vi "Dashboard Main.vi"() -> ()   [LabVIEW 2015]
uses:
  vision/Camera Types.ctl
  <vilib>/Utility/miscctls.llb/LVRowAndColumnTypeDef.ctl
  <vilib>/event_ctls.llb/eventvkey.ctl
  <vilib>/Rock Robotics/WPI/Dashboard/WPI_DashboardLogging Global.vi
  <vilib>/Rock Robotics/Network Tables/NT Read Boolean.vi
  <vilib>/Utility/config.llb/Write Key (String).vi
  <vilib>/Utility/config.llb/Write Key (I32).vi
  <vilib>/Utility/config.llb/NI_LVConfig.lvlib
  Custom/BB_AutonomousSelector.lvlib
  <vilib>/vision/NI_Vision_Development_Module.lvlib
panel:
  in  "Camera Settings":T1={"Frame Rate"=30, "Compression"=30, "Size"=1} {"Frame Rate" scale=1.0..30.0; "Size" items=["640x480", "320x240", "160x120"]}
  in  "DB Camera Config":bool
  out "fps":dbl format="%#.1g"
  out "Mbps":dbl format="%#.1g"
  out "Mbps LED":bool
  out "fps":dbl format="%#.1g"
  out "Mbps 2":dbl format="%#.1g"
  out "Mbps LED 2":bool
  out "Camera Image 2":T2(plugin-control)
  out "Camera Image":T2(plugin-control)
  out "Camera IP 2":string
  in  "TCP":refnum<k5>
  in  "Rec Mode":enum32{"Stop", "Record", "Playback"}(radio)
  in  "Vision":u16(ring) items=["Camera Off", "USB Camera SW", "USB Camera HW", "IP Camera"]
  out "USB Camera IP":string
  out "Image Message":string="Timeout in Camera Communications"
  in  "Dashboard Tab":T3(tab)
  in  "Obstacle":u16(ring) items=["Mars Rock", "BETA_1BALL_STRAIGHT", "BETA_1BALL_CENTER_R", "BETA_2BALL_CENTER_R", "BETA_2BALL_CENTER_L"]
  out "Air Pressure":dbl(knob) scale=0.0..130.0
  in  "Auto Program":u16(ring) items=["Do Nothing", "Drive to Defense", "Breach Defense", "Pure Awesome", "Test Command"]
  in  "Select Auto":string(combo)
  out "NT Connection":bool
  out "Gyro":dbl(knob) scale=0.0..360.0
  out "Mode":T4(ring)=enum."Auto Disabled"
  out "Battery V":dbl
  in  "Robot Start":u16(ring) items=["Mars Rock", "BETA_1BALL_STRAIGHT", "BETA_1BALL_CENTER_R", "BETA_2BALL_CENTER_R", "BETA_2BALL_CENTER_L"]
  out "Connected":bool
  in  "DB/String 9":string
  in  "DB/String 8":string
  in  "DB/String 7":string
  in  "DB/String 6":string
  in  "DB/String 5":string
  in  "DB/String 4":string
  in  "DB/String 3":string
  in  "DB/String 2":string
  in  "DB/String 1":string
  in  "DB/String 0":string
  in  "DB/Slider 0":dbl(slide) scale=0.0..5.0
  in  "DB/Slider 1":dbl(slide) scale=0.0..5.0
  in  "DB/Slider 2":dbl(slide) scale=0.0..5.0
  in  "DB/Slider 3":dbl(slide) scale=0.0..5.0
  out "DB/LED 3":bool
  out "DB/LED 2":bool
  out "DB/LED 1":bool
  out "DB/LED 0":bool
  in  "DB/Button 3":bool
  in  "DB/Button 2":bool
  in  "DB/Button 1":bool
  in  "DB/Button 0":bool caption="New Name"
  in  "LED Color":T5={"Hue"={86.39838557132147, 120.65935737051728}, "Sat"={34.78571428571429, 255.0}, "Val"={91.07142857142858, 255.0}} {"Hue" scale=0.0..255.0 scale format="%#_3g"}
  in  "Test Slider":dbl(slide) scale=0.0..100.0 scale format="%#_3g"
  in  "On/Off":bool caption="Solenoid"
  in  "Test Name":u16(ring) items=["Select the test to run..."]
  in  "Test Tree":string(tree)
  in  "Motor":cluster{"Value":dbl, "Enable":bool} {"Value" scale=-1.0..1.0 scale format="%#_3g"}
  out "Progress":T6 {"Test Progress" scale=0.0..100.0}
  in  "Rev/Fwd":cluster{"Forward":bool, "Reverse":bool}
  in  "Test Ring":u16(ring) items=["Monochrome", "Color"]
  out "Cmd Status":string
  in  "Execute Command":bool
  in  "Command Params":string[][](table)
  in  "Command Selection":i32(listbox)
  in  "CheckList":i32(listbox)
  out "Tree":string(tree)
  out "Background":bool
  # "This tab is a great place for autonomous settings and robot-specific values.\nPlace controls and indicators inside this tab and match name to\nDashboard Variables on robot. You can also delete this comment."
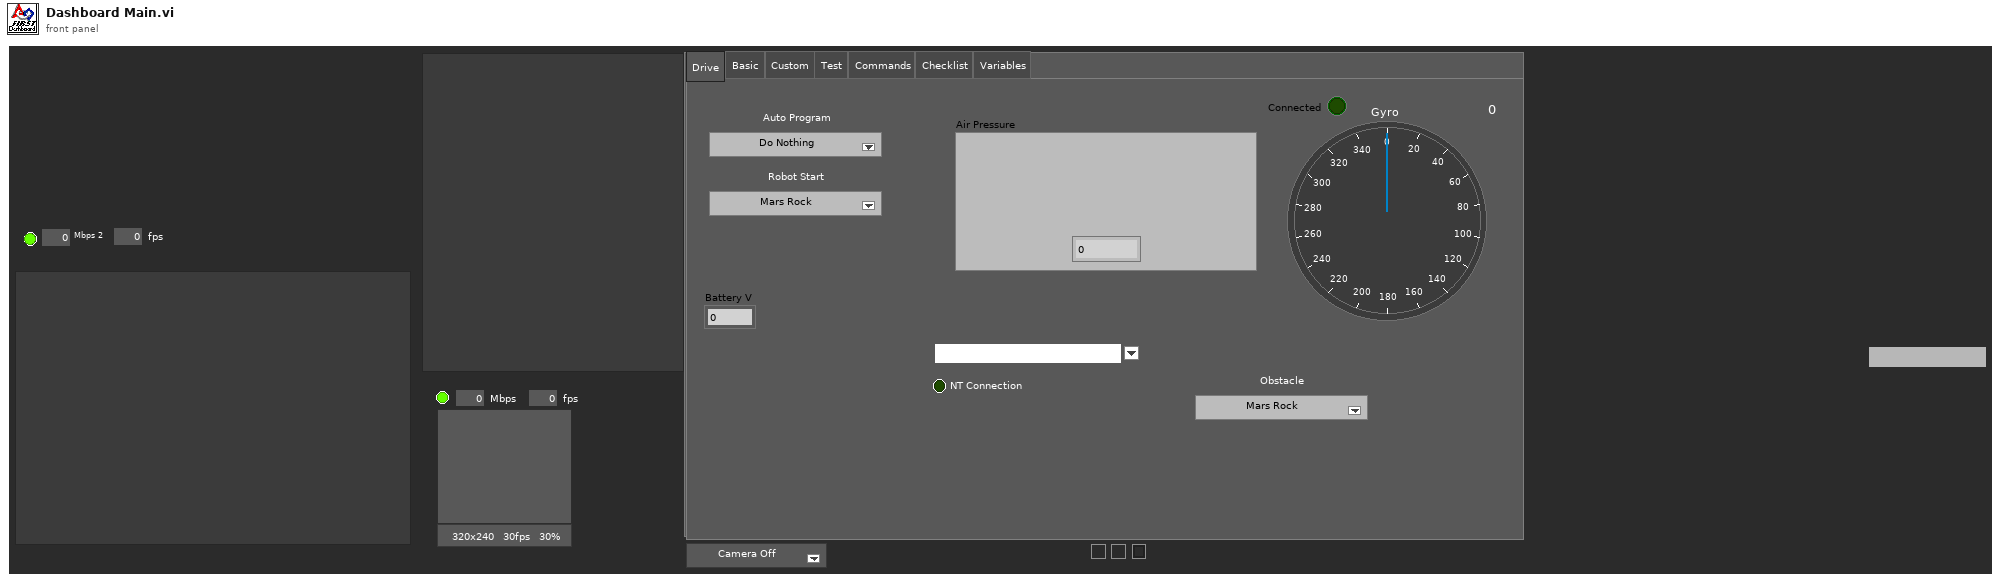
[diagram p1: front panel]
types:
  T1 = cluster{"Frame Rate":i32, "Compression":i32, "Size":u16}
  T2 = typedef "IMAQ Image.ctl" = refnum<image>
  T3 = enum32{"Drive", "Basic", "Custom", "Test", "Commands", "Checklist", "Variables"}
  T4 = enum8{"Tele-Op Disabled", "Tele-Op Enabled", "Auto Disabled", "Auto Enabled", "Test Disabled", "Test Enabled", "Disconnected", "No Code", "E-Stop"}
  T5 = cluster{"Hue":cluster{dbl, dbl}, "Sat":cluster{dbl, dbl}, "Val":cluster{dbl, dbl}}
  T6 = cluster{"Test Progress":u8, "Test Progress Text":string}
  T7 = typedef "Image Type" = u32
  T8 = cluster{"IDs":cluster{"RPC field ID":u16, "Unique ID":u16}, "String":string}
  T9 = enum32{"Drive", "Basic", "Custom", "Test", "Checklist", "Variables"}
  T10 = cluster{void, "Dashboard Tab":refnum<vi>, "Background":refnum<vi>, "Vision":refnum<vi>, "Rec Mode":refnum<vi>, "Test Slider":refnum<vi>, "On/Off ":refnum<vi>, "Test Ring":refnum<vi>, "Rev/Fwd":refnum<vi>, "Test Name":refnum<vi>, "Motor":refnum<vi>, "Progress":refnum<vi>, "CheckList":refnum<vi>, "Tree":refnum<vi>, "Test Tree":refnum<vi>, "Command Params":refnum<vi>, "Command Selection":refnum<vi>, "Execute Command":refnum<vi>, "Cmd Status":refnum<vi>}
  T11 = cluster{"Error Strings":string, "Disable Counts":cluster{u16, u16}, "Rail Faults":cluster{u16, u16, u16}, "Robot IP":string, "DB Mode":u8, "Event Info":cluster{"Name":string, "Type":u8, "Number":u16, "Replay":u8}, "Camera Addr":string}
  T12 = cluster{"Storage":cluster{"Disk Free":u64, "RAM Block":u32, "RAM free":u32}, "CPU Utilization":cluster{"CPU % ISR":sgl, "CPU % Time Crit":sgl, "CPU % Timed Str":sgl, "CPU % High":sgl, "CPU % Above":sgl, "CPU % Normal":sgl, "CPU % Low":sgl}, "CAN":cluster{"% Bus Utilization":sgl, "Bus Off Cnt":u32, "TX_FIFO Full Cnt":u32, "Receive Error Cnt":u8, "Transmit Error Cnt":u8}, "HID":cluster{"HID Outputs":u32, "Rumble Low":u16, "Rumble High":u16}[]}
  T13 = cluster{"Status bits":cluster{"Test Mode":bool, "Autonomous":bool, "Enabled":bool, "Code Start":bool, "Brownout":bool, "Reserved 2":bool, "Reserved 3":bool, "E-Stop":bool}, "Code Trace":cluster{"Disabled":bool, "TeleOp":bool, "Auto":bool, "Test":bool}, "Controller Type":enum16{"unknown", "cRIO", "roboRio"}, "Code?":enum16{"unknown", "noCode", "code"}, "Battery V":dbl}
  T14 = cluster{"Control Bits":cluster{"TestMode":bool, "Autonomous":bool, "Enabled":bool, "FMS Present":bool, bool, bool, bool, "E-Stop":bool}, "Team Station ":u8, "Countdown":sgl, "Joystick Values":cluster{"Axes":dbl[], "Buttons":bool[], "POVs":i16[]}[]}
  T15 = typedef "NI_LVConfig.lvlib/Config Data RefNum.ctl" = refnum<k1>
  T16 = cluster{"Operation":enum16{"Update", "Clear"}, "Color Box":u32}[]
  T17 = typedef "eventvkey.ctl" = enum16{"ASCII", "Enter", "Return", "Shift", "Ctrl", "Alt", "Cmd", "Opt", "Caps", "NumLock", "Clear", "Break", "Up", "Down", "Left", "Right", "Insert", "Delete", "Home", "End", "PageUp", "PageDown", "Escape", "Help", "Pause", "ScrollLock", "F1", "F2", "F3", "F4", "F5", "F6", "F7", "F8", "F9", "F10", "F11", "F12", "F13", "F14", "F15", "F16", "F17", "F18", "F19", "F20", "F21", "F22", "F23", "F24", "Play", "VolumeUp", "VolumeDown", "Mute", "Two Byte Char"}
  T18 = cluster{"Image Size":bool, "Image Type":bool, "Pixel Value":bool, "ROI Information":bool, "Zoom Factor":bool}
  T19 = enum8{"Enabled", "Disabled", "Disabled and Grayed Out"}
  T20 = cluster{"Operation":enum16{"Update", "Clear"}, "Color Box":u32}
  T21 = typedef "LVRowAndColumnTypeDef.ctl" = cluster{"Row":i32, "Column":i32}
  T22 = cluster{"Shift":bool, "Ctrl":bool, "Alt":bool, "Cmd":bool, "Opt":bool}
  T23 = typedef "Camera Types.ctl" = enum16{"206", "1011", "1013", "MS HD3000 square", "MS HD3000 640x480"}
  T24 = cluster{"Distance (ft)":dbl, "Center":cluster{dbl, dbl}, "Normalized Rect":cluster{"Numeric":dbl, "Numeric 2":dbl, "Numeric 3":dbl, "Numeric 5":dbl}}[]
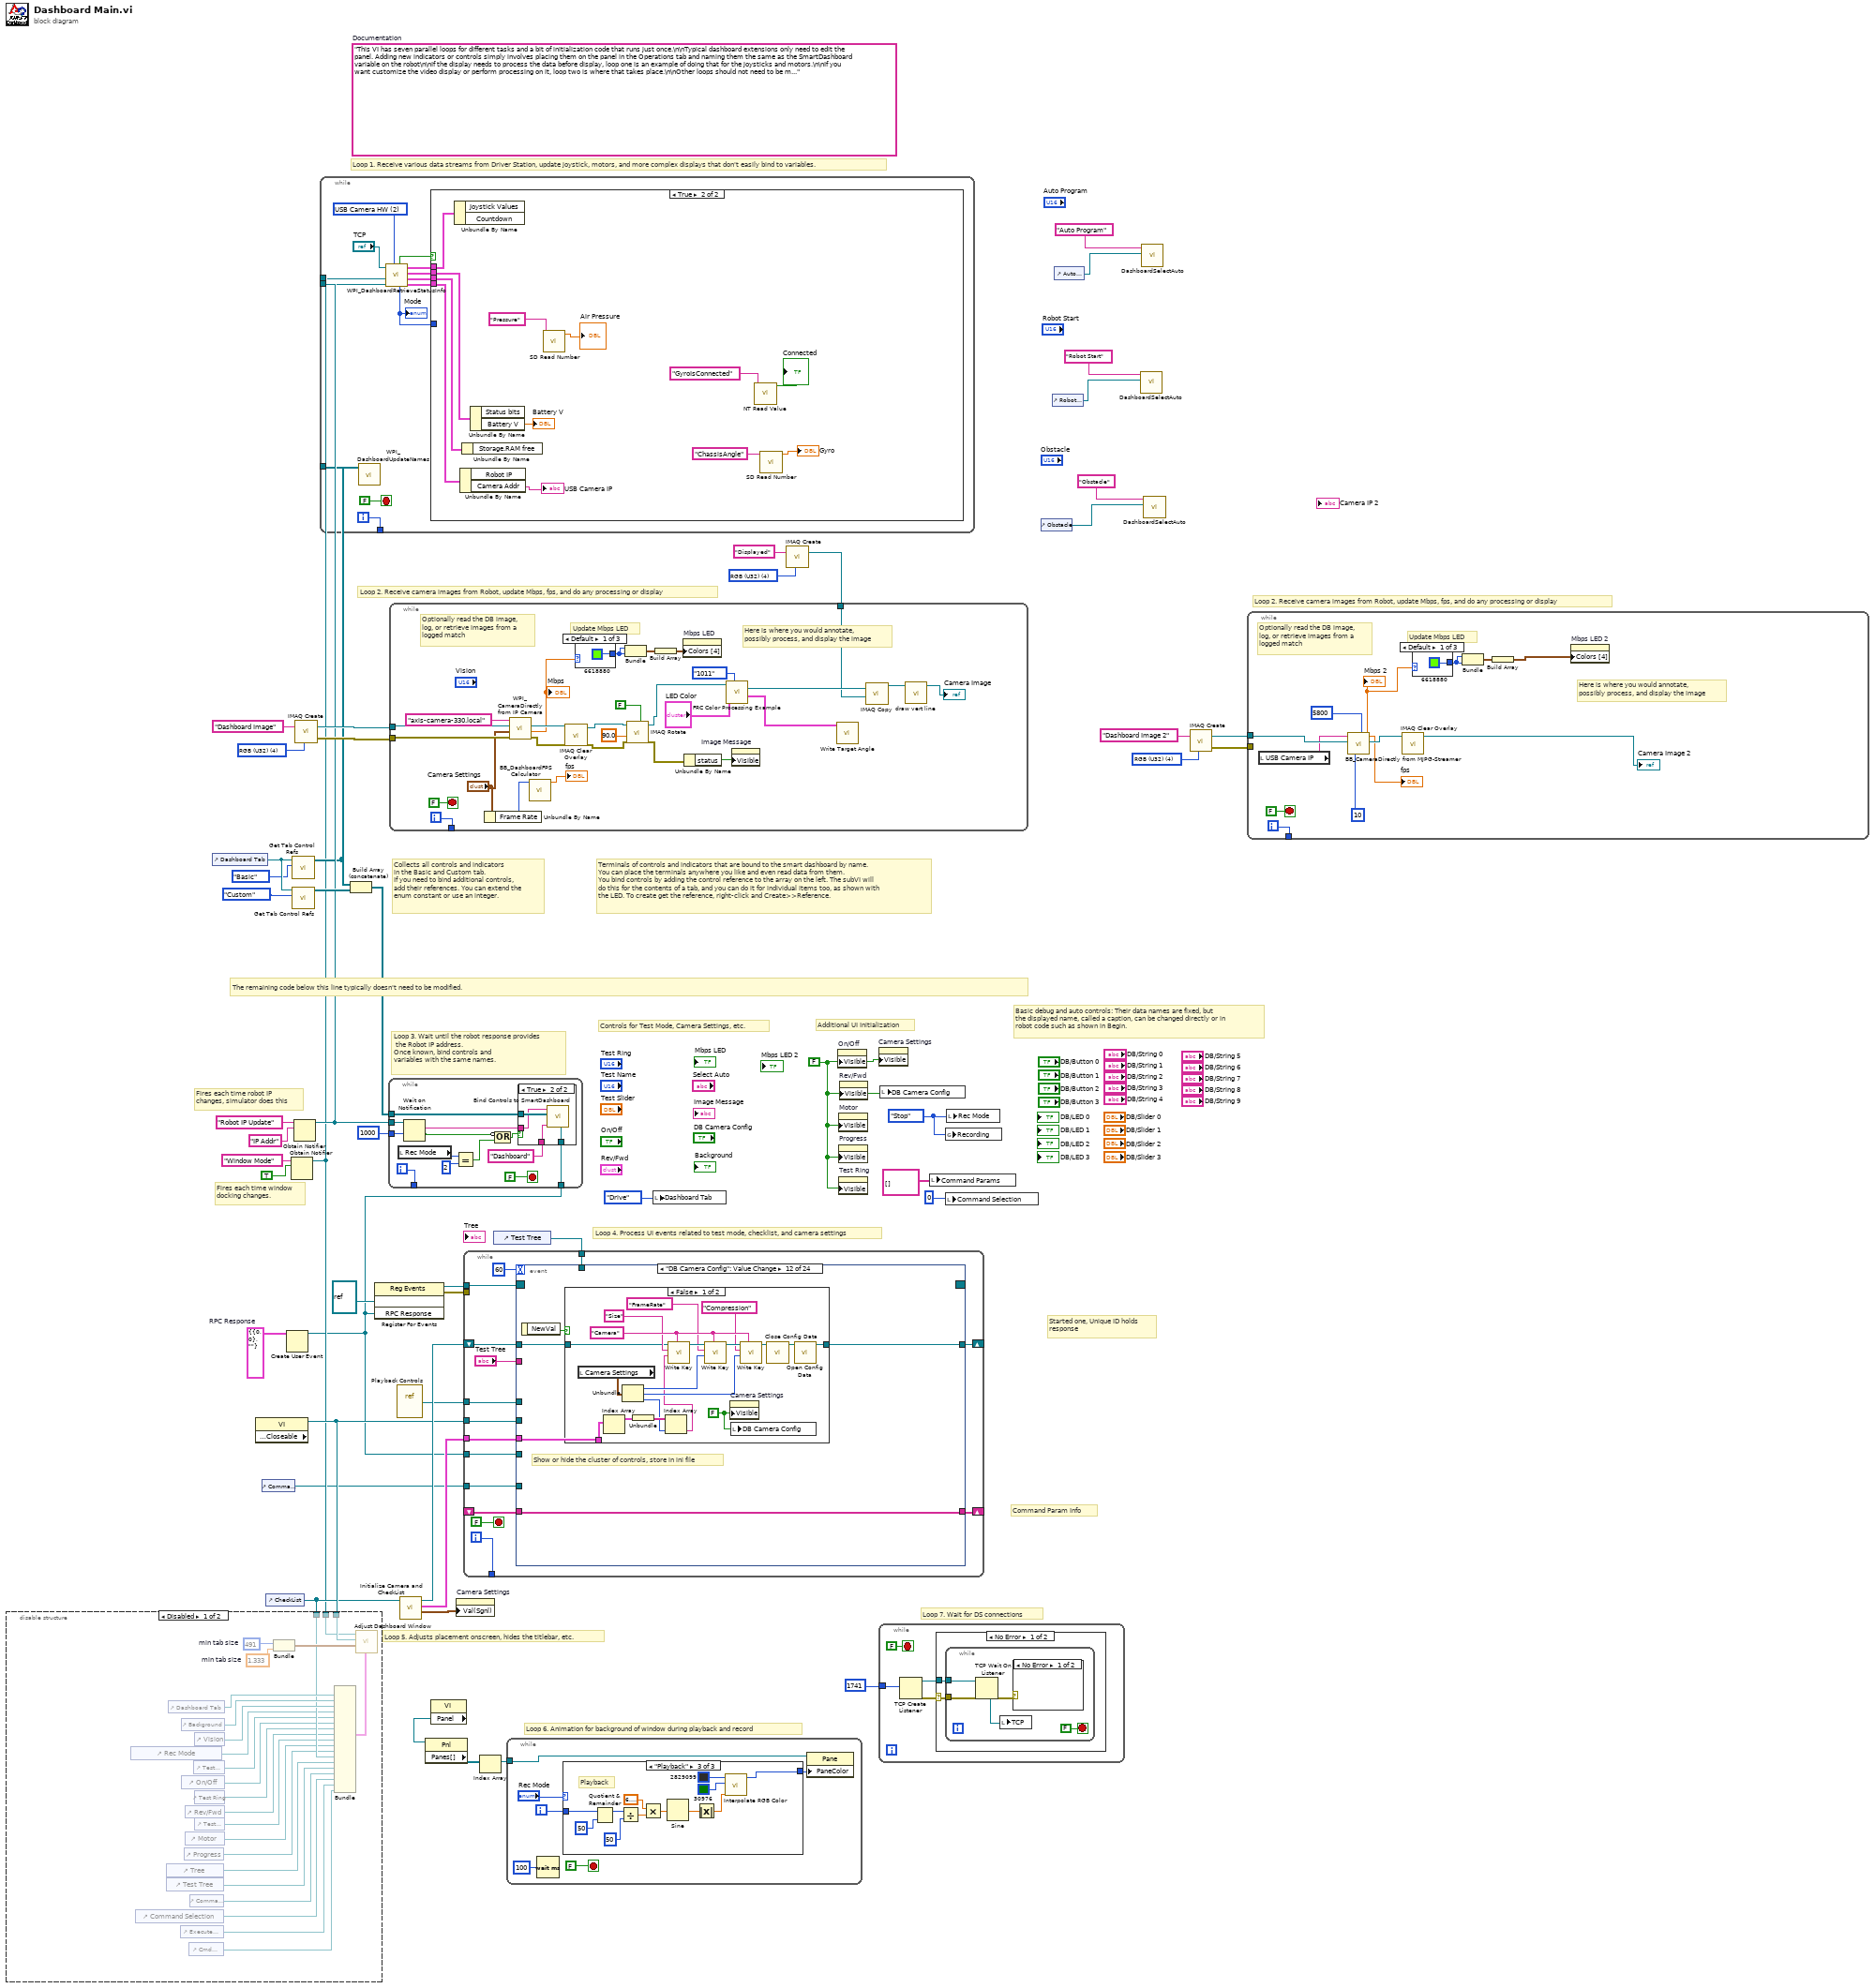
[diagram p0: block diagram]
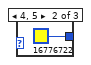
[diagram p3: hidden frame]
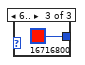
[diagram p4: hidden frame]
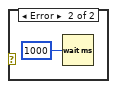
[diagram p5: hidden frame]
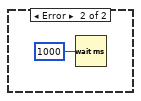
[diagram p6: hidden frame]
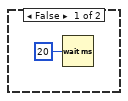
[diagram p7: hidden frame]
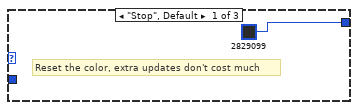
[diagram p8: hidden frame]
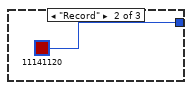
[diagram p9: hidden frame]
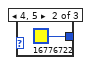
[diagram p11: hidden frame]
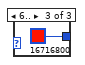
[diagram p12: hidden frame]
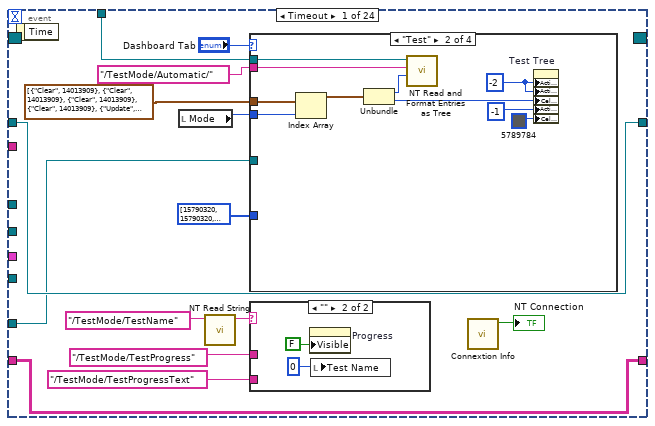
[diagram p13: hidden frame]
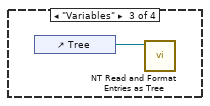
[diagram p15: hidden frame]
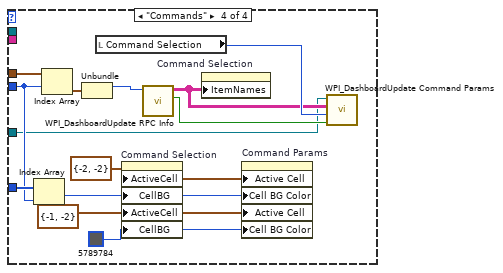
[diagram p16: hidden frame]
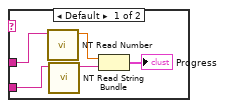
[diagram p17: hidden frame]
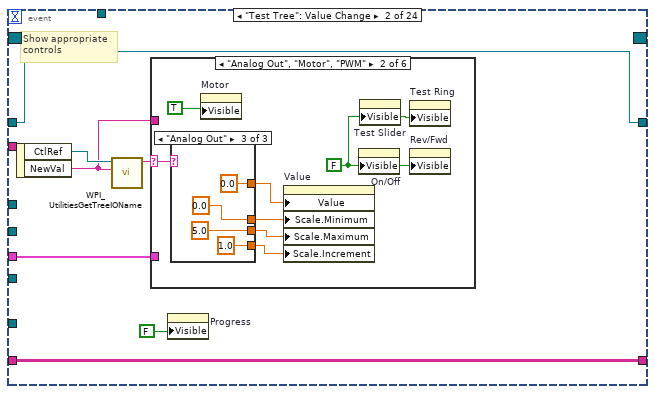
[diagram p18: hidden frame]
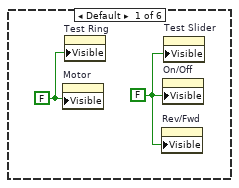
[diagram p19: hidden frame]
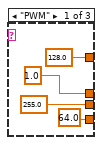
[diagram p20: hidden frame]
diagram:
  w2 = T7 4 items=["Grayscale (U8)", "Grayscale (I16)", "Grayscale (SGL)", "Complex (CSG)", "RGB (U32)", "HSL (U32)", "RGB (U64)"] ("Image Type")
  w7 = T7 4 items=["Grayscale (U8)", "Grayscale (I16)", "Grayscale (SGL)", "Complex (CSG)", "RGB (U32)", "HSL (U32)", "RGB (U64)"] ("Image Type")
  w18 = T8 {"IDs"={"RPC field ID"=0, "Unique ID"=0}, "String"=""}  # RPC Response
  w32 = enum32{"Stop", "Record", "Playback"}."Stop" ("Rec Mode")
  w24 = FALSE ("Visible")
  (unwired) "This VI has seven parallel loops for different tasks and a bit of initialization code that runs just once.\n\nTypical dashboard extensions only need to edit the panel. Adding new indicators or controls simply involves placing them on the panel in the Operations tab and naming them the same as the SmartDashboard variable on the robot\n\nIf the display needs to process the data before display, loop one is an example of doing that for the joysticks and motors.\n\nIf you want customize the video display or perform processing on it, loop two is where that takes place.\n\nOther loops should not need to be modified. They are pretty standard, and document the task they perform."  # Documentation
  w52 = T7 4 items=["Grayscale (U8)", "Grayscale (I16)", "Grayscale (SGL)", "Complex (CSG)", "RGB (U32)", "HSL (U32)", "RGB (U64)"] ("Image Type")
  # "Loop 2. Receive camera images from Robot, update Mbps, fps, and do any processing or display"
  # "Command Param Info"
  # "Started one, Unique ID holds\nresponse"
  # "Loop 7. Wait for DS connections"
  # "Basic debug and auto controls: Their data names are fixed, but\nthe displayed name, called a caption, can be changed directly or in\nrobot code such as shown in Begin."
  # "Controls for Test Mode, Camera Settings, etc."
  # "Additional UI Initialization"
  # "Loop 6. Animation for background of window during playback and record"
  # "Fires each time robot IP\nchanges, simulator does this"
  # "Fires each time window\ndocking changes."
  # "Collects all controls and indicators\nin the Basic and Custom tab.\nIf you need to bind additional controls,\nadd their references. You can extend the\nenum constant or use an integer."
  # "The remaining code below this line typically doesn't need to be modified."
  # "Loop 4. Process UI events related to test mode, checklist, and camera settings"
  # "Terminals of controls and indicators that are bound to the smart dashboard by name.\nYou can place the terminals anywhere you like and even read data from them.\nYou bind controls by adding the control reference to the array on the left. The subVI will\ndo this for the contents of a tab, and you can do it for individual items too, as shown with\nthe LED. To create get the reference, right-click and Create>>Reference."
  # "Loop 3. Wait until the robot response provides\n the Robot IP address.\nOnce known, bind controls and\nvariables with the same names."
  # "Loop 5. Adjusts placement onscreen, hides the titlebar, etc."
  # "Loop 1. Receive various data streams from Driver Station, update joystick, motors, and more complex displays that don't easily bind to variables."
  # "Loop 2. Receive camera images from Robot, update Mbps, fps, and do any processing or display"
  n1 = control-ref of="Dashboard Tab"() -> (w30:refnum<vi>)
  n2 = property class="VI" props=["Front Panel.Closeable"]() -> (reference out=w31:refnum<vi>)  [unwired: 2 in, 2 out]
  n3 = control-ref of="Command Params"() -> (w14:refnum<vi>)
  n4 = control-ref of="CheckList"() -> (w25:refnum<vi>)
  n5 = Create User Event(user event datatype=w18) -> (user event=w15:refnum<user-event>)  [unwired: 1 in, 1 out]
  n6 = Obtain Notifier(name (unnamed)="Window Mode", notification data type=TRUE) -> (notifier out=w21:refnum<notifier>)  [unwired: 2 in, 2 out]
  n7 = disable-structure shown="Disabled" {
    disable-tunnel: w31 -> [w77 _]
    disable-tunnel: w25 -> [w68 _]
    disable-tunnel: w21 -> [w57 _]
    frame Disabled {
      w73 = 491  # min tab size
      w72 = 1.333  # min tab size
      n8 = control-ref of="Rec Mode"() -> (w63:refnum<vi>)
      n9 = control-ref of="Command Selection"() -> (w54:refnum<vi>)
      n10 = control-ref of="Tree"() -> (w67:refnum<vi>)
      n11 = control-ref of="Test Tree"() -> (w66:refnum<vi>)
      n12 = control-ref of="Dashboard Tab"() -> (w75:refnum<vi>)
      n13 = control-ref of="Execute Command"() -> (w55:refnum<vi>)
      n14 = control-ref of="Background"() -> (w70:refnum<vi>)
      n15 = control-ref of="On/Off"() -> (w61:refnum<vi>)
      n16 = control-ref of="Progress"() -> (w58:refnum<vi>)
      n17 = control-ref of="Rev/Fwd"() -> (w59:refnum<vi>)
      n18 = control-ref of="Motor"() -> (w64:refnum<vi>)
      n19 = control-ref of="Cmd Status"() -> (w53:refnum<vi>)
      n20 = control-ref of="Command Params"() -> (w56:refnum<vi>)
      n21 = control-ref of="Test Slider"() -> (w62:refnum<vi>)
      n22 = control-ref of="Vision"() -> (w74:refnum<vi>)
      n23 = control-ref of="Test Ring"() -> (w60:refnum<vi>)
      n24 = control-ref of="Test Name"() -> (w65:refnum<vi>)
      n25 = Bundle("min tab size"=w73, "min tab size"=w72) -> (w71:cluster{"min tab size":i32, "min tab size":dbl})  [unwired: 1 in]
      n26 = Bundle("Dashboard Tab"=w75, "Background"=w70, "Vision"=w74, "Rec Mode"=w63, "Test Slider"=w62, "On/Off"=w61, "Test Ring"=w60, "Rev/Fwd"=w59, "Test Name"=w65, "Motor"=w64, "Progress"=w58, "CheckList"=w68, "Tree"=w67, "Test Tree"=w66, "Command Params"=w56, "Command Selection"=w54, "Execute Command"=w55, "Cmd Status"=w53) -> (w69:T10, w76)  [unwired: 1 in]
      n27 = call "Adjust Dashboard Window.vi"("Sizing Refnums"=w69, "Size Constraints"=w71, "VI"=w77, "WIn Mode"=w57) -> ()  [unwired: 8 in]
    }
    frame Enabled {
    }
  }
  n28 = call <vilib>:"Get Tab Control Refs.vi"("Page Index"=T9."Basic" ("Dashboard Tab"), "TabControl in"=w30) -> ("ControlsOnPage"=w22:refnum<vi>[])  [unwired: 9 in]
  n29 = call <vilib>:"Get Tab Control Refs.vi"("Page Index"=T9."Custom" ("Dashboard Tab"), "TabControl in"=w30) -> ("ControlsOnPage"=w29:refnum<vi>[])  [unwired: 9 in]
  n30 = Obtain Notifier(name (unnamed)="Robot IP Update", notification data type="IP Addr" ("name (unnamed)")) -> (notifier out=w23:refnum<notifier>)  [unwired: 2 in, 2 out]
  n31 = call "IMAQ Create"("Image Name"="Dashboard Image", "Image Type"=w52) -> ("New Image"=w50:T2, "error out"=w49:errorcluster)  [unwired: 2 in, 1 out]
  n32 = while {
    tunnel: [w89] -> _
    tunnel: w23 -> [w83]
    tunnel: w22 -> [w82]
    tunnel: w21 -> [w79]
    i -> [w89]
    stop <- FALSE stop-if-true
    w78 = u16 2 items=["Camera Off", "USB Camera SW", "USB Camera HW", "IP Camera"] ("Vision")
    n33 = call <vilib>:"WPI_DashboardUpdateNames.vi"("Controls on Tab"=w82) -> ()  [unwired: 11 in]
    n34 = call <vilib>:"WPI_DashboardRetrieveStatusInfo.vi"("Vision"=w78, "Binding Refnum"=w83, "Window Mode Notifier"=w79, "TCP Cnx"="TCP") -> ("Power and Errors"=w84:T11, "Robot Metrics"=w87:T12, "Status Info"=w88:T13, "Control Info"=w85:T14, "Robot Mode"=w81:T4, "Process?"=w86:bool)  [unwired: 2 in]
    "Mode" <- w81
    n35 = case shown="True" w86 {
      tunnel: w88 -> [_ w103]
      tunnel: w87 -> [_ w102]
      tunnel: w85 -> [_ w101]
      tunnel: w84 -> [_ w100]
      tunnel: w81 -> [_ _]
      frame False {
        n36 = Wait (ms)(milliseconds to wait=u32 20) -> ()  [unwired: 1 out]
      }
      frame True {
        n37 = Unbundle By Name(w101) -> ()  [unwired: 2 out]
        n38 = Unbundle By Name(w100) -> ("Camera Addr"=→"USB Camera IP":string)  [unwired: 1 out]
        n39 = Unbundle By Name(w102) -> ()  [unwired: 1 out]
        n40 = Unbundle By Name(w103) -> ("Battery V"=→"Battery V":dbl)  [unwired: 1 out]
        n41 = call <vilib>:"SD Read Number.vi"("Name"="Pressure") -> ("Numeric"=→"Air Pressure":dbl)  [unwired: 8 in, 2 out]
        n42 = call-poly <vilib>:"NT Read Value.vi"("Name"="GyroIsConnected") -> ("Boolean"=→"Connected":bool)  [unwired: 9 in, 1 out]
        n43 = call <vilib>:"SD Read Number.vi"("Name"="ChassisAngle") -> ("Numeric"=→"Gyro":dbl)  [unwired: 8 in, 2 out]
      }
    }
  }
  n44 = Build Array (concatenate)(w22, w29) -> (w28:refnum<vi>[])
  n45 = register-events(refnum<vi> refnum, w15) -> (reference out=w36:refnum<event-registration>, error out=w35:errorcluster)  [unwired: 2 in]
  n46 = while {
    tunnel: w28 -> [w116]
    tunnel: w23 -> [w114]
    tunnel: [w112] -> _
    tunnel: u32 1000 ("milliseconds to wait") -> [w111]
    tunnel: w15 -> [w104]
    i -> [w112]
    stop <- FALSE stop-if-true
    n47 = local read "Rec Mode"() -> (w107:enum32{"Stop", "Record", "Playback"})
    n48 = Wait on Notification(notifier=w114, timeout in ms (-1)=w111) -> (notification=w113:string, timed out?=w109:bool)  [unwired: 2 in, 2 out]
    n49 = Equal?(x=w107, y=u16 2 ("Rec Mode")) -> (x = y?=w108:bool)
    n50 = Compound Arithmetic op=OR(invert w109, w108) -> (w110:bool)
    n51 = case shown="True" w110 {
      tunnel: w116 -> [_ w120]
      tunnel: w113 -> [_ w119]
      tunnel: "Dashboard" -> [_ w118]
      tunnel: w104 -> [_ w117]
      frame False {
      }
      frame True {
        n52 = call <vilib>:"Bind Controls to SmartDashboard.vi"("RPC ref"=w117, "Client Name"=w118, "Bound Control Refs"=w120, "Server IP Address"=w119) -> ()  [unwired: 8 in]
      }
    }
  }
  n53 = vi-ref "Playback Controls.vi"() -> (w37:refnum<vi>)
  n54 = call "Initialize Camera and CheckList.vi"("ListBox in"=w25) -> ("Cluster"=w43:cluster{"value":i32, "value":i32, "index":i32}, "Array"=w44:cluster{string[]}[], "File Refnum"=w42:T15)  [unwired: 8 in]
  n55 = property class="VI"() -> ("Panel"=w39:refnum<vi>)  [unwired: 2 in, 2 out]
  n56 = property class="Pnl"(reference=w39) -> ("Panes[]"=w40:refnum<vi>[])  [unwired: 1 in, 2 out]
  n57 = property on="Camera Settings" class="Clust (strict)"("Val(Sgnl)"=w43) -> ()  [unwired: 2 in, 2 out]
  n58 = Index Array(array=w40) -> (element=w38:refnum<vi>)  [unwired: 1 in]
  n59 = control-ref of="Test Tree"() -> (w41:refnum<vi>)
  n60 = while {
    tunnel: w44 -> [w132]
    shift-right: [w131] -> _
    shift-left: w42 -> [w130]
    tunnel: [w129] -> _
    tunnel: w41 -> [w128]
    tunnel: w37 -> [w127]
    tunnel: w36 -> [w126]
    tunnel: w35 -> [_]
    tunnel: w31 -> [w125]
    tunnel: w15 -> [w124]
    tunnel: w14 -> [w123]
    shift-right: [w122] -> _
    shift-left: _ -> [w121]
    i -> [w129]
    stop <- FALSE stop-if-true
    n61 = event shown="[11] \"DB Camera Config\": Value Change" {
      selector: w126 -> [_ _ _ _ _ _ _ _ _ _ _ _ _ _ _ _ _ _ _ _ _ _ _ _]
      dyn-events: [_ _ _ _ _ _ _ _ _ _ _ _ _ _ _ _ _ _ w439 _ _ _ _ _] -> _
      timeout: u32 60 ("milliseconds to wait") -> [_ _ _ _ _ _ _ _ _ _ _ _ _ _ _ _ _ _ _ _ _ _ _ _]
      tunnel: w128 -> [w145 _ _ _ _ _ _ _ _ _ _ _ _ _ _ _ _ _ _ _ _ _ _ _]
      tunnel: "Test Tree" -> [_ _ _ _ _ _ _ _ _ _ _ _ _ w404 w413 w416 w421 w430 _ _ _ _ _ _]
      tunnel: w132 -> [_ w183 _ _ _ _ _ _ _ _ _ w366 w397 _ _ _ _ _ _ _ _ _ _ _]
      tunnel: [w142 w182 w286 w292 w302 w306 w312 w324 w332 w338 w351 w365 w390 w403 w411 w415 w420 w429 w441 w457 w459 w467 w478 w483] -> w131
      tunnel: w130 -> [w142 w182 w286 w292 w302 w306 w312 w324 w332 w338 w351 w364 w390 w403 w411 w415 w420 w429 w441 w457 w459 w467 w478 w483]
      tunnel: w127 -> [_ _ _ _ _ _ _ _ _ _ _ _ _ _ _ _ _ _ w442 _ w462 _ _ _]
      tunnel: w125 -> [_ _ _ _ _ _ _ _ _ _ _ _ _ _ _ _ _ _ w437 _ _ _ _ _]
      tunnel: w124 -> [_ _ _ _ _ _ _ _ _ _ _ _ _ _ _ _ _ _ w435 _ _ _ _ _]
      tunnel: w123 -> [w137 _ _ _ _ _ w310 _ _ _ _ _ _ _ _ _ _ _ _ _ _ _ _ _]
      tunnel: [w136 w181 w285 w291 w301 w307 w308 w318 w329 w337 w350 w363 w389 w402 w410 w414 w419 w428 w434 w455 w458 w463 w471 w484] -> w122
      tunnel: w121 -> [w136 w181 w285 w291 w301 w307 w308 _ _ w337 w350 w363 w389 w402 w410 w414 w419 w428 w434 w455 w458 w463 w471 w484]
      event Timeout {
        n62 = event-data() -> ()  [unwired: 1 in, 1 out]
        n63 = local read "Mode"() -> (w139:T4)
        n64 = call <vilib>:"NT Read String.vi"("Name"="/TestMode/TestName") -> ("String"=w148:string)  [unwired: 9 in, 1 out]
        n65 = case shown="\"Test\"" "Dashboard Tab" {
          tunnel: w145 -> [_ w159 _ _]
          tunnel: "/TestMode/Automatic/" ("Name Pattern") -> [_ w158 _ _]
          tunnel: T16 [{"Operation"=enum."Clear", "Color Box"=14013909}, {"Operation"=enum."Clear", "Color Box"=14013909}, {"Operation"=enum."Clear", "Color Box"=14013909}, {"Operation"=enum."Clear", "Color Box"=14013909}, {"Operation"=enum."Update", "Color Box"=14013909}, {"Operation"=enum."Update", "Color Box"=16777215}, {"Operation"=enum."Clear", "Color Box"=14013909}, {"Operation"=enum."Clear", "Color Box"=14013909}, {"Operation"=enum."Clear", "Color Box"=14013909}] -> [_ w151 _ w168]
          tunnel: w139 -> [_ w150 _ w167]
          tunnel: u32[] [15790320, 15790320, 15790320, 15790320, 16777215, 16777215, 15790320, 15790320, 15790320] -> [_ _ _ w173]
          tunnel: w137 -> [_ _ _ w161]
          frame "Custom", Default {
          }
          frame "Test" {
            w157 = -2 ("Active Item:Row Number")
            n66 = Index Array(array=w151, index=w150) -> (element=w152:T20)
            n67 = Unbundle(w152) -> ("Operation"=w153:enum16{"Update", "Clear"}, "Color Box"=w154:u32)
            n68 = call <vilib>:"NT Read and Format Entries as Tree.vi"("Operation"=w153, "Name Pattern"=w158, "Tree Refnum"=w159) -> ()  [unwired: 7 in, 2 out]
            n69 = property on="Test Tree" class="Tree (strict)"("Active Item Row Number"=w157, "ActiveColNum"=w157, "CellBG"=w154, "Active Item Row Number"=-1 ("Active Item:Row Number"), "CellBG"=u32 5789784 ("Color Box")) -> ()  [unwired: 2 in, 2 out]
          }
          frame "Variables" {
            n70 = control-ref of="Tree"() -> (w160:refnum<vi>)
            n71 = call <vilib>:"NT Read and Format Entries as Tree.vi"("Tree Refnum"=w160) -> ()  [unwired: 9 in, 2 out]
          }
          frame "Commands" {
            w169 = u32 5789784 ("Color Box")
            w170 = T21 {"Row"=-1, "Column"=-2} ("Active Cell:Active Cell")
            w172 = T21 {"Row"=-2, "Column"=-2} ("Active Cell:Active Cell")
            n72 = Index Array(array=w173, index=w167) -> (element=w171:u32)
            n73 = Index Array(array=w168, index=w167) -> (element=w166:T20)
            n74 = Unbundle(w166) -> ("Operation"=w165:enum16{"Update", "Clear"})  [unwired: 1 out]
            n75 = local read "Command Selection"() -> (w164:i32)
            n76 = property on="Command Selection" class="MCListbox (strict)"("ActiveCell"=w172, "CellBG"=w171, "ActiveCell"=w170, "CellBG"=w169) -> ()  [unwired: 2 in, 2 out]
            n77 = call <vilib>:"WPI_DashboardUpdate RPC Info.vi"("Operation"=w165) -> ("update"=w163:bool, "commands"=w162:string[][])  [unwired: 9 in]
            n78 = property on="Command Selection" class="MCListbox (strict)"("ItemNames"=w162) -> ()  [unwired: 2 in, 2 out]
            n79 = property on="Command Params" class="Tbl (strict)"("Active Cell"=w172, "Cell BG Color"=w171, "Active Cell"=w170, "Cell BG Color"=w169) -> ()  [unwired: 2 in, 2 out]
            n80 = call <vilib>:"WPI_DashboardUpdate Command Params.vi"("Update"=w163, "NewVal"=w164, "Commands"=w162, "Param Tbl"=w161) -> ()  [unwired: 7 in, 1 out]
          }
        }
        n81 = case shown="\"\"" w148 {
          tunnel: "/TestMode/TestProgress" ("Name") -> [w175 _]
          tunnel: "/TestMode/TestProgressText" ("Name") -> [w174 _]
          frame Default {
            n82 = call <vilib>:"NT Read Number.vi"("Name"=w175) -> ("Numeric"=w176:dbl)  [unwired: 9 in, 1 out]
            n83 = call <vilib>:"NT Read String.vi"("Name"=w174) -> ("String"=w177:string)  [unwired: 9 in, 1 out]
            n84 = Bundle("Numeric"=w176, "String"=w177) -> (→"Progress":cluster{"Numeric":dbl, "String":string})  [unwired: 1 in]
          }
          frame "" {
            n85 = property on="Progress" class="Clust (strict)"("Visible"=FALSE) -> ()  [unwired: 2 in, 2 out]
            n86 = local write "Test Name"(u16 0) -> ()
          }
        }
        n87 = call <vilib>:"Connextion Info.vi"() -> ("Connected"=→"NT Connection":bool)  [unwired: 10 in, 1 out]
      }
      event "Test Tree": Value Change {
        # "Show appropriate\ncontrols"
        n88 = event-data() -> ("CtlRef"=w186:refnum<vi>, "NewVal"=w184:string)  [unwired: 1 in]
        n89 = call <vilib>:"WPI_UtilitiesGetTreeIOName.vi"("NewVal"=w184, "TreeControl in"=w186) -> ("I/O Name"=w187:string)  [unwired: 9 in]
        n90 = case shown="\"Analog Out\", \"Motor\", \"PWM\"" w187 {
          selector: w187 -> [_ w194 _ w216 w225 _]
          tunnel: w184 -> [_ _ w213 w215 _ w232]
          tunnel: w183 -> [_ _ _ _ _ w231]
          frame Default {
            w189 = FALSE ("Visible")
            w188 = FALSE ("Visible")
            n91 = property on="Motor" class="Clust (strict)"("Visible"=w188) -> ()  [unwired: 2 in, 2 out]
            n92 = property on="Test Ring" class="Ring (strict)"("Visible"=w188) -> ()  [unwired: 2 in, 2 out]
            n93 = property on="Rev/Fwd" class="Clust (strict)"("Visible"=w189) -> ()  [unwired: 2 in, 2 out]
            n94 = property on="On/Off" class="Bool (strict)"("Visible"=w189) -> ()  [unwired: 2 in, 2 out]
            n95 = property on="Test Slider" class="Slide (strict)"("Visible"=w189) -> ()  [unwired: 2 in, 2 out]
          }
          frame "Analog Out", "Motor", "PWM" {
            w195 = FALSE ("Visible")
            n96 = case shown="\"Analog Out\"" w194 {
              tunnel: [1.0 ("Value") -1.0 ("Value") 0.0 ("Value")] -> w193
              tunnel: [255.0 ("Value") 1.0 ("Value") 5.0 ("Value")] -> w192
              tunnel: [128.0 ("Value") 0.0 ("Value") 0.0 ("Value")] -> w191
              tunnel: [64.0 ("Value") 0.5 ("Value") 1.0 ("Value")] -> w190
              frame "PWM" {
              }
              frame "Motor", Default {
              }
              frame "Analog Out" {
              }
            }
            n97 = property on="Motor" class="Clust (strict)"("Visible"=TRUE) -> ()  [unwired: 2 in, 2 out]
            n98 = property on="Value" class="Slide (strict)"("Value"=w191, "Scale.Minimum"=w193, "Scale.Maximum"=w192, "Scale.Increment"=w190) -> ()  [unwired: 2 in, 2 out]
            n99 = property on="On/Off" class="Bool (strict)"("Visible"=w195) -> ()  [unwired: 2 in, 2 out]
            n100 = property on="Test Slider" class="Slide (strict)"("Visible"=w195) -> ()  [unwired: 2 in, 2 out]
            n101 = property on="Test Ring" class="Ring (strict)"("Visible"=w195) -> ()  [unwired: 2 in, 2 out]
            n102 = property on="Rev/Fwd" class="Clust (strict)"("Visible"=w195) -> ()  [unwired: 2 in, 2 out]
          }
          frame "Servo" {
            w211 = FALSE ("Visible")
            n103 = call <vilib>:"NT Read Number.vi"("Name"=w213) -> ("Numeric"=w212:dbl)  [unwired: 9 in, 1 out]
            n104 = property on="Test Slider" class="Slide (strict)"("Visible"=TRUE, "Scale.Maximum"=170.0 ("Scale.Range:Maximum")) -> ()  [unwired: 2 in, 2 out]
            n105 = local write "Test Slider"(w212) -> ()
            n106 = property on="Motor" class="Clust (strict)"("Visible"=w211) -> ()  [unwired: 2 in, 2 out]
            n107 = property on="Rev/Fwd" class="Clust (strict)"("Visible"=w211) -> ()  [unwired: 2 in, 2 out]
            n108 = property on="On/Off" class="Bool (strict)"("Visible"=w211) -> ()  [unwired: 2 in, 2 out]
            n109 = property on="Test Ring" class="Ring (strict)"("Visible"=w211) -> ()  [unwired: 2 in, 2 out]
          }
          frame "Relay", "Solenoid" {
            w214 = FALSE ("Visible")
            n110 = property on="Motor" class="Clust (strict)"("Visible"=w214) -> ()  [unwired: 2 in, 2 out]
            n111 = property on="Test Slider" class="Slide (strict)"("Visible"=w214) -> ()  [unwired: 2 in, 2 out]
            n112 = Search and Replace String(input string=w215, search string="/Value  **", replace string="/Direction") -> (result string=w221:string)  [unwired: 5 in, 3 out]
            n113 = property on="Test Ring" class="Ring (strict)"("Visible"=w214) -> ()  [unwired: 2 in, 2 out]
            n114 = call <vilib>:"NT Read String.vi"("Name"=w221) -> ("String"=w219:string)  [unwired: 9 in, 1 out]
            n115 = Equal?(x="Both directions", y=w219) -> (x = y?=w217:bool)
            n116 = Not(x=w217) -> (.not. x?=w218:bool)
            n117 = property on="Rev/Fwd" class="Clust (strict)"("Visible"=w217) -> ()  [unwired: 2 in, 2 out]
            n118 = property on="On/Off" class="Bool (strict)"("Visible"=w218, "Caption.Text"=w216) -> ()  [unwired: 2 in, 2 out]
          }
          frame "Compressor", "Digital Out" {
            w224 = FALSE ("Visible")
            # "Get direction and finish"
            n119 = property on="Motor" class="Clust (strict)"("Visible"=w224) -> ()  [unwired: 2 in, 2 out]
            n120 = property on="Test Slider" class="Slide (strict)"("Visible"=w224) -> ()  [unwired: 2 in, 2 out]
            n121 = property on="Test Ring" class="Ring (strict)"("Visible"=w224) -> ()  [unwired: 2 in, 2 out]
            n122 = property on="On/Off" class="Bool (strict)"("Visible"=TRUE, "Caption.Text"=w225) -> ()  [unwired: 2 in, 2 out]
            n123 = property on="Rev/Fwd" class="Clust (strict)"("Visible"=FALSE) -> ()  [unwired: 2 in, 2 out]
          }
          frame "Camera" {
            n124 = call <vilib>:"Get Last Path Segment.vi"("String in"=w232) -> ("String out"=w233:string)  [unwired: 10 in]
            n125 = property on="On/Off" class="Bool (strict)"("Visible"=FALSE) -> ()  [unwired: 2 in, 2 out]
            n126 = property on="Motor" class="Clust (strict)"("Visible"=FALSE) -> ()  [unwired: 2 in, 2 out]
            n127 = property on="Rev/Fwd" class="Clust (strict)"("Visible"=FALSE) -> ()  [unwired: 2 in, 2 out]
            n128 = case shown="\"White Balance  **\"" w233 {
              tunnel: w232 -> [w239 w248 w257 w266 w275 _ w281]
              tunnel: w231 -> [w237 w245 w254 w263 w272 _ _]
              frame "Size  **" {
                n129 = Index Array(array=w237) -> (element=w236:cluster{string[]})  [unwired: 1 in]
                n130 = call <vilib>:"NT Read String.vi"("Name"=w239) -> ("String"=w238:string)  [unwired: 9 in, 1 out]
                n131 = Unbundle(w236) -> (w234:string[])
                n132 = Match First String(2:w234, 3:w238) -> (0:w235:i32)  [unwired: 1 out]
                n133 = property on="Test Ring" class="Ring (strict)"("Value"=w235, "Strings []"=w234) -> ()  [unwired: 2 in, 2 out]
                n134 = property on="Test Ring" class="Ring (strict)"("Visible"=TRUE) -> ()  [unwired: 2 in, 2 out]
                n135 = property on="Test Slider" class="Slide (strict)"("Visible"=FALSE) -> ()  [unwired: 2 in, 2 out]
              }
              frame "White Balance  **" {
                n136 = Index Array(array=w245, index=1) -> (element=w246:cluster{string[]})
                n137 = call <vilib>:"NT Read String.vi"("Name"=w248) -> ("String"=w247:string)  [unwired: 9 in, 1 out]
                n138 = Unbundle(w246) -> (w243:string[])
                n139 = Match First String(2:w243, 3:w247) -> (0:w242:i32)  [unwired: 1 out]
                n140 = property on="Test Ring" class="Ring (strict)"("Value"=w242, "Strings []"=w243) -> ()  [unwired: 2 in, 2 out]
                n141 = property on="Test Ring" class="Ring (strict)"("Visible"=TRUE) -> ()  [unwired: 2 in, 2 out]
                n142 = property on="Test Slider" class="Slide (strict)"("Visible"=FALSE) -> ()  [unwired: 2 in, 2 out]
              }
              frame "Exposure  **" {
                n143 = Index Array(array=w254, index=2) -> (element=w255:cluster{string[]})
                n144 = call <vilib>:"NT Read String.vi"("Name"=w257) -> ("String"=w256:string)  [unwired: 9 in, 1 out]
                n145 = Unbundle(w255) -> (w251:string[])
                n146 = Match First String(2:w251, 3:w256) -> (0:w252:i32)  [unwired: 1 out]
                n147 = property on="Test Ring" class="Ring (strict)"("Value"=w252, "Strings []"=w251) -> ()  [unwired: 2 in, 2 out]
                n148 = property on="Test Ring" class="Ring (strict)"("Visible"=TRUE) -> ()  [unwired: 2 in, 2 out]
                n149 = property on="Test Slider" class="Slide (strict)"("Visible"=FALSE) -> ()  [unwired: 2 in, 2 out]
              }
              frame "Exposure Priority  **" {
                n150 = Index Array(array=w263, index=3) -> (element=w264:cluster{string[]})
                n151 = call <vilib>:"NT Read String.vi"("Name"=w266) -> ("String"=w265:string)  [unwired: 9 in, 1 out]
                n152 = Unbundle(w264) -> (w260:string[])
                n153 = Match First String(2:w260, 3:w265) -> (0:w261:i32)  [unwired: 1 out]
                n154 = property on="Test Ring" class="Ring (strict)"("Value"=w261, "Strings []"=w260) -> ()  [unwired: 2 in, 2 out]
                n155 = property on="Test Ring" class="Ring (strict)"("Visible"=TRUE) -> ()  [unwired: 2 in, 2 out]
                n156 = property on="Test Slider" class="Slide (strict)"("Visible"=FALSE) -> ()  [unwired: 2 in, 2 out]
              }
              frame "Color Enable  **" {
                n157 = Index Array(array=w272, index=4) -> (element=w273:cluster{string[]})
                n158 = call <vilib>:"NT Read String.vi"("Name"=w275) -> ("String"=w274:string)  [unwired: 9 in, 1 out]
                n159 = Unbundle(w273) -> (w269:string[])
                n160 = Match First String(2:w269, 3:w274) -> (0:w270:i32)  [unwired: 1 out]
                n161 = property on="Test Ring" class="Ring (strict)"("Value"=w270, "Strings []"=w269) -> ()  [unwired: 2 in, 2 out]
                n162 = property on="Test Ring" class="Ring (strict)"("Visible"=TRUE) -> ()  [unwired: 2 in, 2 out]
                n163 = property on="Test Slider" class="Slide (strict)"("Visible"=FALSE) -> ()  [unwired: 2 in, 2 out]
              }
              frame Default {
                n164 = property on="Test Ring" class="Ring (strict)"("Visible"=FALSE) -> ()  [unwired: 2 in, 2 out]
                n165 = property on="Test Slider" class="Slide (strict)"("Visible"=FALSE) -> ()  [unwired: 2 in, 2 out]
              }
              frame "Brightness  **", "Color Level  **", "Compression  **", "FPS  **", "Sharpness  **" {
                n166 = call <vilib>:"NT Read Number.vi"("Name"=w281) -> ("Numeric"=w280:dbl)  [unwired: 9 in, 1 out]
                n167 = local write "Test Slider"(w280) -> ()
                n168 = property on="Test Slider" class="Slide (strict)"("Visible"=TRUE, "Scale.Maximum"=100.0 ("Scale.Range:Maximum")) -> ()  [unwired: 2 in, 2 out]
                n169 = property on="Test Ring" class="Ring (strict)"("Visible"=FALSE) -> ()  [unwired: 2 in, 2 out]
              }
            }
          }
        }
        n170 = property on="Progress" class="Clust (strict)"("Visible"=FALSE) -> ()  [unwired: 2 in, 2 out]
      }
      event "Test Name": Mouse Enter {
        # "Populate the ring with the list of tests"
        n171 = event-data() -> ()  [unwired: 1 in, 1 out]
        n172 = call <vilib>:"NT Read String Array.vi"("Name"="/TestMode/TestList") -> ("String Array"=w290:string[])  [unwired: 9 in, 1 out]
        n173 = Build Array (concatenate)("Select the test to run...", w290) -> (w289:string[])
        n174 = property on="Test Name" class="Ring (strict)"("Strings []"=w289) -> ()  [unwired: 2 in, 2 out]
      }
      event "Test Name": Value Change {
        w293 = FALSE ("Visible")
        # "Tell the robot the test name to run"
        n175 = event-data() -> ("NewVal"=w297:u16)  [unwired: 1 in]
        n176 = property on="Test Name" class="Ring (strict)"() -> ("Strings []"=w298:string[])  [unwired: 2 in, 2 out]
        n177 = local write "Progress"(T6 {"Test Progress"=0, "Test Progress Text"=""} ("Progress")) -> ()
        n178 = Index Array(array=w298, index=w297) -> (element=w296:string)
        n179 = call <vilib>:"NT Write String.vi"("String"=w296, "Name"="/TestMode/TestName") -> ()  [unwired: 9 in, 1 out]
        n180 = property on="Progress" class="Clust (strict)"("Visible"=TRUE) -> ()  [unwired: 2 in, 2 out]
        n181 = property on="Motor" class="Clust (strict)"("Visible"=w293) -> ()  [unwired: 2 in, 2 out]
        n182 = property on="Test Slider" class="Slide (strict)"("Visible"=w293) -> ()  [unwired: 2 in, 2 out]
        n183 = property on="On/Off" class="Bool (strict)"("Visible"=w293) -> ()  [unwired: 2 in, 2 out]
        n184 = property on="Rev/Fwd" class="Clust (strict)"("Visible"=w293) -> ()  [unwired: 2 in, 2 out]
        n185 = property on="Test Ring" class="Ring (strict)"("Visible"=w293) -> ()  [unwired: 2 in, 2 out]
      }
      event "Select Auto": Mouse Enter {
        # "Populate the combo box with the list of autonomous options"
        n186 = event-data() -> ()  [unwired: 1 in, 1 out]
        n187 = call <vilib>:"NT Read String Array.vi"("Name"="Auto List") -> ("String Array"=w300:string[])  [unwired: 9 in, 1 out]
        n188 = property on="Select Auto" class="CmbBox"("Strings[]"=w300) -> ()  [unwired: 2 in, 2 out]
      }
      event "Select Auto": Value Change {
        # "User modified the Auto Selection. Write to NT variable so robot knows."
        n189 = event-data() -> ("NewVal"=w304:string)  [unwired: 1 in]
        n190 = call <vilib>:"NT Write String.vi"("String"=w304, "Name"="Auto Selector") -> ()  [unwired: 9 in, 1 out]
      }
      event "Command Selection": Value Change {
        # "Get the params and show in table"
        n191 = event-data() -> ("NewVal"=w311:i32)  [unwired: 1 in]
        n192 = property on="Command Selection" class="MCListbox (strict)"() -> ("ItemNames"=w309:string[][])  [unwired: 2 in, 2 out]
        n193 = call <vilib>:"WPI_DashboardUpdate Command Params.vi"("NewVal"=w311, "Commands"=w309, "Param Tbl"=w310) -> ()  [unwired: 8 in, 1 out]
      }
      event "Execute Command": Value Change {
        # "Started one, Unique ID holds\nresponse"
        n194 = event-data() -> ()  [unwired: 1 in, 1 out]
        n195 = property on="Command Selection" class="MCListbox (strict)"() -> ("ItemNames"=w323:string[][])  [unwired: 2 in, 2 out]
        n196 = Index Array(array=w323, index (row)="Command Selection", index (col)=0) -> (element=w321:string)
        n197 = call <vilib>:"Invoke Commands.vi"("Command Params"="Command Params", "Function Name"=w321) -> ("Params"=w317:u8, "Started"=w316:bool)  [unwired: 7 in, 1 out]
        n198 = Array Subset(array="Command Params", length (row)=w317) -> (w318:string[][])  [unwired: 3 in]
        n199 = Select(t="Executing" ("Cmd Status"), s=w316, f="" ("Cmd Status")) -> (s? t:f=→"Cmd Status":string)
      }
      event "Command Selection": Double Click {
        n200 = event-data() -> ("Row"=w333:i32)  [unwired: 1 in]
        n201 = property on="Command Selection" class="MCListbox (strict)"() -> ("ItemNames"=w336:string[][])  [unwired: 2 in, 2 out]
        n202 = local read "Command Params"() -> (w331:string[][])
        n203 = Index Array(array=w336, index (row)=w333, index (col)=0) -> (element=w334:string)
        n204 = call <vilib>:"Invoke Commands.vi"("Command Params"=w331, "Function Name"=w334) -> ("Params"=w330:u8, "Started"=w325:bool)  [unwired: 7 in, 1 out]
        n205 = Array Subset(array=w331, length (row)=w330) -> (w329:string[][])  [unwired: 3 in]
        n206 = Select(t="Executing" ("Cmd Status"), s=w325, f="" ("Cmd Status")) -> (s? t:f=w326:string)
        n207 = local write "Cmd Status"(w326) -> ()
      }
      event "CheckList": Double Click {
        # "Shift clears all"
        # "Update symbols on the listbox"
        n208 = event-data() -> ("PlatMods.Shift"=w339:bool, "Row"=w341:i32)  [unwired: 1 in]
        n209 = case shown="True" w339 {
          tunnel: w341 -> [w345 _]
          tunnel: 1 -> [w344 _]
          frame False {
            n210 = property on="CheckList" class="LstBox (strict)"() -> ("Item Symbols"=w343:i32[])  [unwired: 2 in, 2 out]
            n211 = Replace Array Subset(array=w343, new element=w344, index=w345) -> (w342:i32[])
            n212 = property on="CheckList" class="LstBox (strict)"("Item Symbols"=w342) -> ()  [unwired: 2 in, 2 out]
          }
          frame True {
            w346 = 0 ("Top Row")
            n213 = property on="CheckList" class="LstBox (strict)"() -> ("Number of Rows"=w348:u32)  [unwired: 2 in, 2 out]
            n214 = Initialize Array(0, w348) -> (w347:i32[])
            n215 = property on="CheckList" class="LstBox (strict)"("Top Row"=w346, "Value"=w346, "Item Symbols"=w347) -> ()  [unwired: 2 in, 2 out]
          }
        }
      }
      event "CheckList": Key Down {
        # "Update symbols on the listbox\nLeft and right keys check and uncheck"
        n216 = event-data() -> ("VKey"=w353:T17)  [unwired: 1 in]
        n217 = case shown="\"Left\", \"Right\"" w353 {
          selector: w353 -> [w358 _]
          tunnel: eventvkey."Left" ("VKey") -> [w356 _]
          frame "Left", "Right" {
            n218 = Equal?(x=w356, y=w358) -> (x = y?=w357:bool)
            n219 = Select(t=0, s=w357, f=1) -> (s? t:f=w359:i32)
            n220 = property on="CheckList" class="LstBox (strict)"() -> ("Item Symbols"=w362:i32[])  [unwired: 2 in, 2 out]
            n221 = Replace Array Subset(array=w362, new element=w359, index="CheckList") -> (w361:i32[])
            n222 = property on="CheckList" class="LstBox (strict)"("Item Symbols"=w361) -> ()  [unwired: 2 in, 2 out]
          }
          frame Default {
          }
        }
      }
      event "DB Camera Config": Value Change {
        # "Show or hide the cluster of controls, store in ini file"
        n223 = event-data() -> ("NewVal"=w367:bool)  [unwired: 1 in]
        n224 = case shown="False" w367 {
          tunnel: w366 -> [w376 _]
          tunnel: [w369 w387] -> w365
          tunnel: w364 -> [w368 w387]
          frame False {
            w383 = "Camera"
            w386 = FALSE ("Visible")
            n225 = local read "Camera Settings"() -> (w375:T1)
            n226 = Index Array(array=w376) -> (element=w379:cluster{string[]})  [unwired: 1 in]
            n227 = Unbundle(w375) -> ("Frame Rate"=w374:i32, "Compression"=w373:i32, "Size"=w377:u16)
            n228 = Unbundle(w379) -> (w378:string[])
            n229 = Index Array(array=w378, index=w377) -> (element=w372:string)
            n230 = call-poly <vilib>:"Write Key.vi"("section"=w383, "value"=w372, "key"="Size", "refnum"=w368) -> ("refnum out"=w385:T15)  [unwired: 2 in, 5 out]
            n231 = call-poly <vilib>:"Write Key.vi"("section"=w383, "value"=w374, "key"="FrameRate", "refnum"=w385) -> ("refnum out"=w384:T15)  [unwired: 1 in, 6 out]
            n232 = property on="Camera Settings" class="Clust (strict)"("Visible"=w386) -> ()  [unwired: 2 in, 2 out]
            n233 = local write "DB Camera Config"(w386) -> ()
            n234 = call-poly <vilib>:"Write Key.vi"("section"=w383, "value"=w373, "key"="Compression", "refnum"=w384) -> ("refnum out"=w370:T15)  [unwired: 1 in, 6 out]
            n235 = call <vilib>:"Close Config Data.vi"("refnum"=w370) -> ("file path"=w371:path)  [unwired: 2 in, 8 out]
            n236 = call <vilib>:"Open Config Data.vi"("configuration file path"=w371) -> ("refnum"=w369:T15)  [unwired: 8 in, 2 out]
          }
          frame True {
            n237 = property on="Camera Settings" class="Clust (strict)"("Visible"=TRUE) -> ()  [unwired: 2 in, 2 out]
          }
        }
      }
      event "Camera Settings": Value Change {
        # "Update summary string when any elements of DB camera change"
        n238 = event-data() -> ("NewVal"=w401:T1)  [unwired: 1 in]
        n239 = Index Array(array=w397) -> (element=w396:cluster{string[]})  [unwired: 1 in]
        n240 = Unbundle(w401) -> ("Frame Rate"=w392:i32, "Compression"=w391:i32, "Size"=w394:u16)
        n241 = Unbundle(w396) -> (w395:string[])
        n242 = Index Array(array=w395, index=w394) -> (element=w393:string)
        n243 = Format Into String(format string="%s   %dfps   %d%%", w393, w392, w391) -> (resulting string=w398:string)  [unwired: 2 in, 1 out]
        n244 = Build Array(w398) -> (w399:string[])
        n245 = property on="DB Camera Config" class="Bool (strict)"("Strings [4]"=w399) -> ()  [unwired: 2 in, 2 out]
      }
      event "Motor.Enable": Value Change {
        # "When the test mode otor enable helper is set, update that\ntree row item's value"
        n246 = event-data() -> ("NewVal"=w408:bool)  [unwired: 1 in]
        n247 = Unbundle("Motor") -> ("Value"=w407:dbl)  [unwired: 1 out]
        n248 = Select(t=w407, s=w408, f=0.0) -> (s? t:f=w405:dbl)
        n249 = call <vilib>:"NT Write Number.vi"("Numeric"=w405, "Name"=w404) -> ()  [unwired: 9 in, 1 out]
      }
      event "Test Slider": Value Change {
        # "When the test mode slider helper is set, update that\ntree row item's value"
        n250 = event-data() -> ("NewVal"=w412:dbl)  [unwired: 1 in]
        n251 = call <vilib>:"NT Write Number.vi"("Numeric"=w412, "Name"=w413) -> ()  [unwired: 9 in, 1 out]
      }
      event "On/Off": Value Change {
        # "When the test mode on/off helper value is set, update that\ntree row item's value"
        n252 = event-data() -> ("NewVal"=w418:bool)  [unwired: 1 in]
        n253 = Boolean To (0,1)(Boolean=w418) -> (0, 1=w417:i16)
        n254 = call <vilib>:"NT Write Number.vi"("Numeric"=w417, "Name"=w416) -> ()  [unwired: 9 in, 1 out]
      }
      event "Rev/Fwd": Value Change {
        # "When the test mode helper value for relays is set, update that\ntree row item's value"
        n255 = event-data() -> ("NewVal.Forward"=w427:bool, "NewVal.Reverse"=w426:bool)  [unwired: 1 in]
        n256 = Boolean To (0,1)(Boolean=w427) -> (0, 1=w423:i16)
        n257 = Boolean To (0,1)(Boolean=w426) -> (0, 1=w425:i16)
        n258 = Negate(x=w425) -> (-x=w424:i16)
        n259 = Add(x=w423, y=w424) -> (x+y=w422:i16)
        n260 = call <vilib>:"NT Write Number.vi"("Numeric"=w422, "Name"=w421) -> ()  [unwired: 9 in, 1 out]
      }
      event "Test Ring": Value Change {
        # "When a test mode helper value is selected from the ring,\nset the tree item's variable to the string value"
        n261 = event-data() -> ("NewVal"=w432:u16)  [unwired: 1 in]
        n262 = property on="Test Ring" class="Ring (strict)"() -> ("Strings []"=w433:string[])  [unwired: 2 in, 2 out]
        n263 = Index Array(array=w433, index=w432) -> (element=w431:string)
        n264 = call <vilib>:"NT Write String.vi"("String"=w431, "Name"=w430) -> ()  [unwired: 9 in, 1 out]
      }
      event "Rec Mode": Value Change {
        # "Update globals for recording mode and path to read log from.\nClear when logging and let NetworkTables set path for vision to\nuse."
        n265 = event-data() -> ("NewVal"=w443:enum32{"Stop", "Record", "Playback"})  [unwired: 1 in]
        n266 = global write "WPI_DashboardLogging Global.vi" "Logging Filename"(path "") -> ()
        n267 = global write "WPI_DashboardLogging Global.vi" "Recording"(w443) -> ()
        n268 = case shown="\"Playback\"" w443 {
          tunnel: w442 -> [_ w445 w454]
          tunnel: [_ _ w453] -> w439
          tunnel: [_ _ w452] -> _
          tunnel: w437 -> [_ _ w450]
          tunnel: cluster{i32, i32} {-250, 170} -> [_ _ w449]
          tunnel: [_ _ T18 {"Image Size"=TRUE, "Image Type"=TRUE, "Pixel Value"=TRUE, "ROI Information"=TRUE, "Zoom Factor"=FALSE} ("Image Information Shown:All Elements")] -> _
          tunnel: [_ _ TRUE ("Zoom Factor")] -> _
          tunnel: w435 -> [_ _ w446]
          frame Default {
          }
          frame "Stop", "Record" {
            # "Place Window too"
            n269 = invoke class="VI" method="FP.Close"(reference=w445) -> (reference out=w444:refnum<vi>)  [unwired: 2 in, 2 out]
            n270 = invoke class="VI" method="Abort VI"(reference=w444) -> ()  [unwired: 2 in, 3 out]
          }
          frame "Playback" {
            n271 = call "Open Playback Panel.vi"("Offset"=w449, "DB VI Ref"=w450, "Playback in"=w454) -> ("Playback out"=w451:refnum<vi>)  [unwired: 8 in]
            n272 = register-events(w451, w446) -> (reference out=w453:refnum<event-registration>, error out=w452:errorcluster)  [unwired: 2 in]
          }
        }
        n273 = call <vilib>:"WPI_DashboardNT Log FieldName Cache.vi"("Operation"=enum16{"Lookup/Add", "Index", "Clear"}."Clear") -> ()  [unwired: 8 in, 3 out]
      }
      event Panel Close {
        w456 = enum32{"Stop", "Record", "Playback"}."Stop" ("Rec Mode")
        # "Playback window has been closed, abort"
        n274 = event-data() -> ()  [unwired: 1 in, 4 out]
        n275 = local write "Rec Mode"(w456) -> ()
        n276 = global write "WPI_DashboardLogging Global.vi" "Recording"(w456) -> ()
      }
      event Panel Close {
        # "Abort playback window and ourself"
        n277 = event-data() -> ()  [unwired: 1 in, 4 out]
        n278 = invoke class="VI" method="FP.Close"(reference=w462) -> (reference out=w461:refnum<vi>)  [unwired: 2 in, 2 out]
        n279 = invoke class="VI" method="Abort VI"(reference=w461) -> (error out=w460:errorcluster)  [unwired: 2 in, 2 out]
        n280 = invoke class="VI" method="Abort VI"(error in=w460) -> ()  [unwired: 2 in, 3 out]
      }
      event User Event {
        n281 = event-data() -> ("IDs"=w470:cluster{"RPC field ID":u16, "Unique ID":u16}, "String"=w469:string)  [unwired: 1 in]
        n282 = Bundle("IDs"=w470, "String"=w469) -> (w468:T8)  [unwired: 1 in]
        n283 = call <vilib>:"Retrieve RPC Response.vi"("RPC Response"=w468) -> ("Output"=w465:string[][])  [unwired: 10 in]
        n284 = Build Array (concatenate)(w463, w465) -> (w464:string[][])
        n285 = local write "Command Params"(w464) -> ()
        n286 = local write "Cmd Status"("" ("Cmd Status")) -> ()
      }
      event "Vision": Value Change {
        # "Enable/Disable Compression slider.\nHW USB is hard-coded into the camera"
        n287 = event-data() -> ("NewVal"=w477:u16)  [unwired: 1 in]
        n288 = Equal?(x=w477, y=u32 2 ("milliseconds to wait")) -> (x = y?=w475:bool)
        n289 = Select(t=T19."Disabled and Grayed Out" ("Disabled"), s=w475, f=T19."Enabled" ("Disabled")) -> (s? t:f=w472:T19)
        n290 = property on="Compression" class="Slide (strict)"("DisabledEnum"=w472) -> ()  [unwired: 2 in, 2 out]
      }
      event "Tree": Double Click {
        n291 = event-data() -> ("PlatMods"=w482:T22, "Tag"=w481:string)  [unwired: 1 in]
        n292 = Unbundle(w482) -> ("Shift"=w480:bool)  [unwired: 4 out]
        n293 = Not(x=w480) -> (.not. x?=w479:bool)
        n294 = call <vilib>:"NT Update Persistence.vi"("Persistence"=w479, "Name"=w481) -> ()  [unwired: 9 in, 1 out]
      }
    }
  }
  n295 = while {
    tunnel: w38 -> [w486]
    i -> [w489]
    stop <- FALSE stop-if-true
    n296 = Wait (ms)(milliseconds to wait=u32 100) -> ()  [unwired: 1 out]
    n297 = case shown="\"Playback\"" "Rec Mode" {
      tunnel: w489 -> [_ _ w504]
      tunnel: [u32 2829099 ("Base Color") u32 11141120 ("Target Color") w493] -> w485
      frame "Stop", Default {
        # "Reset the color, extra updates don't cost much"
      }
      frame "Record" {
      }
      frame "Playback" {
        # "Playback"
        n298 = Quotient & Remainder(x=w504, y=u32 50 ("milliseconds to wait")) -> (x-y*floor(x/y)=w500:u32)  [unwired: 1 out]
        n299 = Divide(x=w500, y=u32 50 ("milliseconds to wait")) -> (x/y=w497:dbl)
        n300 = Multiply(x=6.283185307179586, y=w497) -> (x*y=w502:dbl)
        n301 = Sine(x=w502) -> (sin(x)=w501:dbl)
        n302 = Absolute Value(x=w501) -> (abs(x)=w494:dbl)
        n303 = call "Interpolate RGB Color.vi"("Proportion"=w494, "Target Color"=u32 30976, "Base Color"=u32 2829099) -> ("Result Color"=w493:u32)  [unwired: 8 in]
      }
    }
    n304 = property class="Pane"(reference=w486, "PaneColor"=w485) -> ()  [unwired: 1 in, 2 out]
  }
  n305 = local write "Dashboard Tab"(T3."Drive" ("Dashboard Tab")) -> ()
  n306 = call "IMAQ Create"("Image Name"="Displayed", "Image Type"=w2) -> ("New Image"=w1:T2)  [unwired: 2 in, 2 out]
  n307 = while {
    tunnel: w50 -> [w526]
    tunnel: w49 -> [w525]
    tunnel: [w531] -> _
    tunnel: w1 -> [w509]
    i -> [w531]
    stop <- FALSE stop-if-true
    # "Here is where you would annotate,\npossibly process, and display the image"
    # "Update Mbps LED"
    # "Optionally read the DB image,\nlog, or retrieve images from a\nlogged match"
    n308 = Unbundle By Name("Camera Settings") -> ("Frame Rate"=w519:i32)
    n309 = call <vilib>:"WPI_CameraDirectly from IP Camera.vi"("error in"=w525, "Camera Settings"="Camera Settings", "Image"=w526, "address"="axis-camera-330.local") -> ("error out"=w524:errorcluster, "Bandwidth (Mbps)"=w522:dbl, "Image Out"=w523:T2)  [unwired: 5 in]
    "Mbps" <- w522
    n310 = call "BB_DashboardFPS Calculator.vi"("Average Count"=w519) -> ("fps"=→"fps":dbl)  [unwired: 10 in]
    n311 = call "IMAQ Clear Overlay"("error in (no error)"=w524, "Image"=w523) -> ("error out"=w516:errorcluster, "Image Out"=w518:T2)  [unwired: 1 in, 7 out]
    n312 = case shown="Default" w522 {
      tunnel: [u32 6618880 ("Color Box") u32 16776722 ("Color Box") u32 16716800 ("Color Box")] -> w527
      frame Default {
      }
      frame 4, 5 {
      }
      frame 6.. {
      }
    }
    n313 = Bundle("Color Box"=w527, "Color Box"=w527) -> (w529:cluster{"Color Box":u32, "Color Box":u32})  [unwired: 1 out]
    n314 = call "IMAQ Rotate"("Maintain Size"=FALSE, "error in (no error)"=w516, "Angle (degrees)"=sgl 90.0, "Image Src"=w518) -> ("error out"=w515:errorcluster, "Image Dst Out"=w511:T2)  [unwired: 6 in]
    n315 = Build Array(w529) -> (w528:cluster{"Color Box":u32, "Color Box":u32}[])
    n316 = property on="Mbps LED" class="Bool (strict)"("Colors [4]"=w528) -> ()  [unwired: 2 in, 2 out]
    n317 = Unbundle By Name(w515) -> ("status"=w530:bool)
    n318 = call "FRC Color Processing Example.vi"("Image In"=w511, "LED Color"="LED Color", "Camera Type"=Camera_Types."1011") -> ("Original Image"=w510:T2, "Detected Targets"=w505:T24)  [unwired: 6 in]
    n319 = property on="Image Message" class="Str"("Visible"=w530) -> ()  [unwired: 2 in, 2 out]
    n320 = call "Write Target Angle.vi"("Detected Targets"=w505) -> ()  [unwired: 11 in]
    n321 = call "IMAQ Copy"("Image Dst"=w509, "Image Src"=w510) -> ("Image Dst Out"=w508:T2)  [unwired: 4 in, 1 out]
    n322 = call "draw vert line.vi"("Refnum in"=w508) -> ("Refnum out"=→"Camera Image":T2)  [unwired: 10 in]
  }
  n323 = property on="On/Off" class="Bool (strict)"("Visible"=w24) -> ()  [unwired: 2 in, 2 out]
  n324 = property on="Motor" class="Clust (strict)"("Visible"=w24) -> ()  [unwired: 2 in, 2 out]
  n325 = property on="Progress" class="Clust (strict)"("Visible"=w24) -> ()  [unwired: 2 in, 2 out]
  n326 = property on="Test Ring" class="Ring (strict)"("Visible"=w24) -> ()  [unwired: 2 in, 2 out]
  n327 = property on="Rev/Fwd" class="Clust (strict)"("Visible"=w24) -> ()  [unwired: 2 in, 2 out]
  n328 = property on="Camera Settings" class="Clust (strict)"("Visible"=w24) -> ()  [unwired: 2 in, 2 out]
  n329 = while {
    tunnel: u16 1741 ("timeout ms (25000)") -> [w537]
    stop <- FALSE stop-if-true
    n330 = TCP Create Listener(10:w537) -> (0:w536:errorcluster, 3:w538:refnum<k5>)  [unwired: 4 in, 1 out]
    n331 = case shown="No Error" w536 {
      selector: w536 -> [w540 _]
      tunnel: w538 -> [w541 _]
      frame No Error {
        n332 = while {
          tunnel: w541 -> [w544]
          tunnel: w540 -> [w543]
          stop <- FALSE stop-if-true
          n333 = TCP Wait On Listener(8:w543, 11:w544) -> (0:w545:errorcluster, 4:w546:refnum<k5>)  [unwired: 2 in, 3 out]
          n334 = local write "TCP"(w546) -> ()
          n335 = case shown="No Error" w545 {
            frame No Error {
            }
            frame Error {
              n336 = Wait (ms)(milliseconds to wait=u32 1000) -> ()  [unwired: 1 out]
            }
          }
        }
      }
      frame Error {
        n337 = Wait (ms)(milliseconds to wait=u32 1000) -> ()  [unwired: 1 out]
      }
    }
  }
  n338 = local write "DB Camera Config"(w24) -> ()
  n339 = local write "Command Params"(string[][] [] ("Command Params")) -> ()
  n340 = global write "WPI_DashboardLogging Global.vi" "Recording"(w32) -> ()
  n341 = local write "Command Selection"(u16 0 ("milliseconds to wait")) -> ()
  n342 = local write "Rec Mode"(w32) -> ()
  n343 = control-ref of="Obstacle"() -> (w8:refnum<vi>)
  n344 = control-ref of="Robot Start"() -> (w11:refnum<vi>)
  n345 = control-ref of="Auto Program"() -> (w12:refnum<vi>)
  n346 = call "DashboardSelectAuto.vi"("Table Prefix"="Robot Start", "Autonomous Mode Ring"=w11) -> ()  [unwired: 9 in]
  n347 = call "DashboardSelectAuto.vi"("Table Prefix"="Auto Program", "Autonomous Mode Ring"=w12) -> ()  [unwired: 9 in]
  n348 = call "DashboardSelectAuto.vi"("Table Prefix"="Obstacle", "Autonomous Mode Ring"=w8) -> ()  [unwired: 9 in]
  n349 = call "IMAQ Create"("Image Name"="Dashboard Image 2", "Image Type"=w7) -> ("New Image"=w5:T2, "error out"=w4:errorcluster)  [unwired: 2 in, 1 out]
  n350 = while {
    tunnel: w5 -> [w559]
    tunnel: w4 -> [_]
    tunnel: [w560] -> _
    i -> [w560]
    stop <- FALSE stop-if-true
    # "Here is where you would annotate,\npossibly process, and display the image"
    # "Update Mbps LED"
    # "Optionally read the DB image,\nlog, or retrieve images from a\nlogged match"
    n351 = local read "USB Camera IP"() -> (w557:string)
    n352 = call "BB_CameraDirectly from MJPG-Streamer.vi"("remote port or service name"=u16 5800, "fps"=10, "Image"=w559, "address"=w557) -> ("Bandwidth (Mbps)"=w556:dbl, "Image Out"=w558:T2, "FPS"=→"fps":dbl)  [unwired: 4 in, 1 out]
    "Mbps 2" <- w556
    n353 = call "IMAQ Clear Overlay"("Image"=w558) -> ("Image Out"=→"Camera Image 2":T2)  [unwired: 2 in, 8 out]
    n354 = case shown="Default" w556 {
      tunnel: [u32 6618880 ("Color Box") u32 16776722 ("Color Box") u32 16716800 ("Color Box")] -> w552
      frame Default {
      }
      frame 4, 5 {
      }
      frame 6.. {
      }
    }
    n355 = Bundle("Color Box"=w552, "Color Box"=w552) -> (w554:cluster{"Color Box":u32, "Color Box":u32})  [unwired: 1 out]
    n356 = Build Array(w554) -> (w553:cluster{"Color Box":u32, "Color Box":u32}[])
    n357 = property on="Mbps LED 2" class="Bool (strict)"("Colors [4]"=w553) -> ()  [unwired: 2 in, 2 out]
  }
